vi "WriteBounds.vi"(8 "error in (no error)":errorcluster, 11 "Bounds":T1) -> (0 "error out":errorcluster)   [LabVIEW 2017, in "DisplayWindow.lvlib" / "DisplayWindow.lvclass"]
doc: "Write the boundaries of the DisplayWindow to the configuration file."
uses:
  DisplayWindow.lvclass
  <vilib>/Utility/miscctls.llb/LVRectTypeDef.ctl
  <vilib>/Utility/config.llb/Write Key (I32).vi
  <vilib>/Utility/config.llb/NI_LVConfig.lvlib
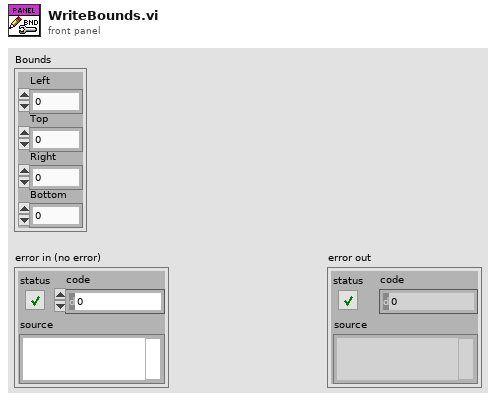
[diagram p1: front panel]
types:
  T1 = typedef "LVRectTypeDef.ctl" = cluster{"Left":i16, "Top":i16, "Right":i16, "Bottom":i16}
  T2 = typedef "NI_LVConfig.lvlib/Config Data RefNum.ctl" = refnum<k1>
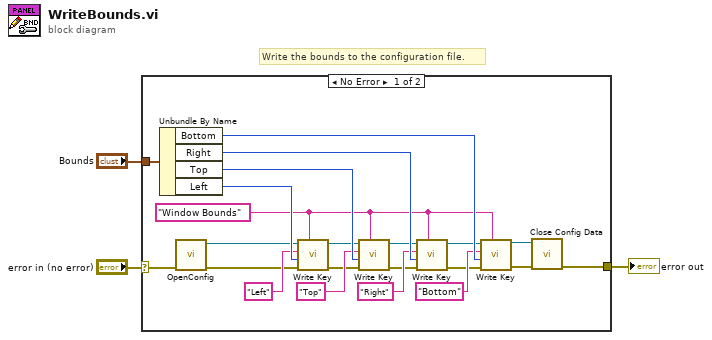
[diagram p0: block diagram]
diagram:
  # "Write the bounds to the configuration file."
  n1 = case shown="No Error" "error in (no error)" {
    selector: "error in (no error)" -> [w21 w26]
    tunnel: [w20 w26] -> w2
    tunnel: "Bounds" -> [w4 _]
    frame No Error {
      w13 = "Window Bounds"
      n2 = Unbundle By Name(w4) -> ("Bottom"=w22:i16, "Right"=w24:i16, "Top"=w23:i16, "Left"=w25:i16)
      n3 = call "OpenConfig.vi"("error in (no error)"=w21) -> ("error out"=w8:errorcluster, "refnum"=w19:T2)  [unwired: 9 in]
      n4 = call-poly <vilib>:"Write Key.vi"("section"=w13, "error in (no error)"=w8, "value"=w25, "key"="Left", "refnum"=w19) -> ("error out"=w7:errorcluster, "refnum out"=w18:T2)  [unwired: 4 in, 1 out]
      n5 = call-poly <vilib>:"Write Key.vi"("section"=w13, "error in (no error)"=w7, "value"=w23, "key"="Top", "refnum"=w18) -> ("error out"=w6:errorcluster, "refnum out"=w17:T2)  [unwired: 4 in, 1 out]
      n6 = call-poly <vilib>:"Write Key.vi"("section"=w13, "error in (no error)"=w6, "value"=w24, "key"="Right", "refnum"=w17) -> ("error out"=w5:errorcluster, "refnum out"=w16:T2)  [unwired: 4 in, 1 out]
      n7 = call-poly <vilib>:"Write Key.vi"("section"=w13, "error in (no error)"=w5, "value"=w22, "key"="Bottom", "refnum"=w16) -> ("error out"=w14:errorcluster, "refnum out"=w15:T2)  [unwired: 4 in, 1 out]
      n8 = call <vilib>:"Close Config Data.vi"("error in (no error)"=w14, "refnum"=w15) -> ("error out"=w20:errorcluster)  [unwired: 8 in, 1 out]
    }
    frame Error {
    }
  }
  "error out" <- w2
